vi "Execute.vi"(8 "error in (no error)":errorcluster, 11 "Node in":refnum<class "bt_WaitOn_Queue.lvclass">) -> (0 "error out":errorcluster, 1 "Status":T1, 3 "Node out":refnum<class "bt_WaitOn_Queue.lvclass">)   [LabVIEW 2021, in "BT.lvlib" / "bt_WaitOn_Queue.lvclass"]
uses:
  bt_WaitOn_Queue.lvclass
  C:/Users/Tim/Documents/GitHub/LV_Behaviour_Tree/Source/Support/Nodes/Leaves/Synch/Parent/WaitOn/bt_WaitOn_Synch.lvclass
  abs_Node/Status.ctl
  bt_WaitOn_Queue.lvclass/bt_WaitOn_Queue.ctl
  abs_Node/bt_Node.lvclass
  Parent/WaitOn/bt_WaitOn_Synch.lvclass
  With Values/WaitOn/bt_WaitOn_Synch_WithValues.lvclass
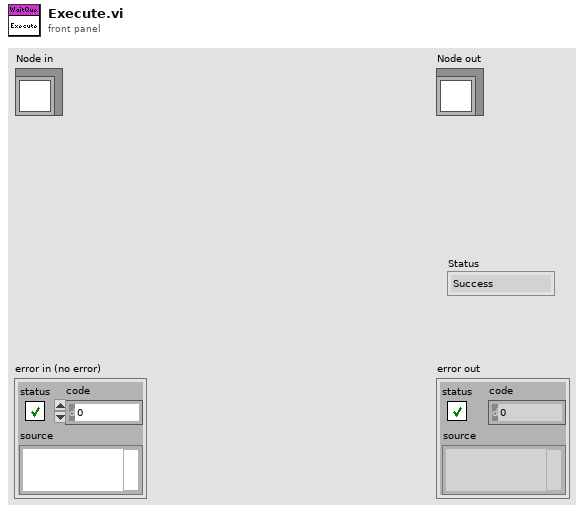
[diagram p1: front panel]
types:
  T1 = typedef "BT.lvlib/bt_Node.lvclass/Status.ctl" = enum16{"Success", "Failure", "Running"}
  T2 = typedef "NI_Data Type.lvlib/Data Type.ctl" = enum8{"Invalid Type", "Void", "I8", "I16", "I32", "I64", "U8", "U16", "U32", "U64", "Single Float", "Double Float", "Extended Float", "Single Complex", "Double Complex", "Extended Complex", "Enum U8", "Enum U16", "Enum U32", "Enum U64", "Single Float With Unit", "Double Float With Unit", "Extended Float With Unit", "Single Complex with Unit", "Double Complex with Unit", "Extended Complex with Unit", "Boolean", "String", "Path", "Picture", "Tag", "Array", "Cluster", "Variant", "LV Variant", "Waveform", "Timestamp", "Digital Waveform", "Digital Data", "ExpressData", "Refnum", "External Data", "VI", "Poly VI", "LabVIEW Class Instance", "Fixed Point", "Set Collection", "Map Collection"}
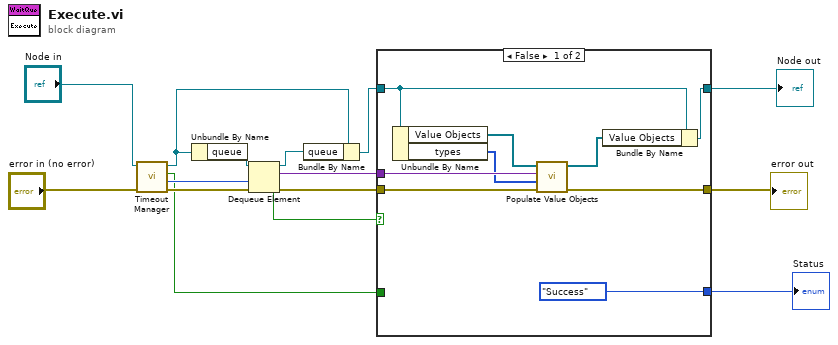
[diagram p0: block diagram]
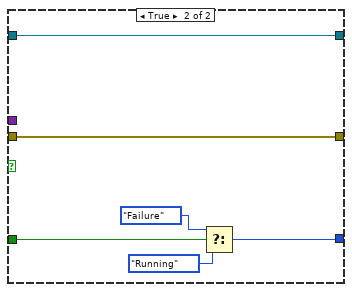
[diagram p2: hidden frame]
diagram:
  n1 = call "Timeout Manager.vi"("error in (no error)"="error in (no error)", "bt_WaitOn_Synch in"="Node in") -> ("error out"=w12:errorcluster, "Timeout"=w9:i32, "Timeout Now?"=w6:bool, "bt_WaitOn_Synch out"=w10:refnum<class "bt_WaitOn_Queue.lvclass">)  [unwired: 6 in]
  n2 = Unbundle By Name(w10) -> ("queue"=w15:refnum<queue>)
  n3 = Dequeue Element(queue=w15, timeout in ms (-1)=w9, error in (no error)=w12) -> (queue out=w14:refnum<queue>, element=w3:variant, timed out?=w8:bool, error out=w7:errorcluster)
  n4 = Bundle By Name(cluster=w10, "queue"=w14) -> (w2:refnum<class "bt_WaitOn_Queue.lvclass">)
  n5 = case shown="False" w8 {
    tunnel: w7 -> [w23 w26]
    tunnel: w6 -> [_ w29]
    tunnel: [Status."Success" ("Status") w27] -> w5
    tunnel: [w22 w26] -> w4
    tunnel: w3 -> [w21 _]
    tunnel: w2 -> [w18 w25]
    tunnel: [w16 w25] -> w1
    frame False {
      n6 = Unbundle By Name(w18) -> ("Value Objects"=w20:refnum<class "Abs_Value.lvclass">[], "types"=w19:T2[])
      n7 = call "Populate Value Objects.vi"("error in (no error)"=w23, "LabVIEW types"=w19, "Variant"=w21, "Value Objects Type"=w20) -> ("error out"=w22:errorcluster, "Value Objects Out"=w17:refnum<class "Abs_Value.lvclass">[])  [unwired: 6 in]
      n8 = Bundle By Name(cluster=w18, "Value Objects"=w17) -> (w16:refnum<class "bt_WaitOn_Queue.lvclass">)
    }
    frame True {
      n9 = Select(t=Status."Failure" ("Status"), s=w29, f=Status."Running") -> (s? t:f=w27:T1)
    }
  }
  "error out" <- w4
  "Node out" <- w1
  "Status" <- w5
